vi "拉压判定.vi"(7 "Result":refnum<vi>, 10 "判定参数":T2, 11 "XY曲线":cluster{"X":dbl[], "Y":dbl[]}[](array[cluster])) -> (2 "大小":i32, 3 "OK？":bool)   [LabVIEW 2020]
panel:
  in  "最大值判定":T1
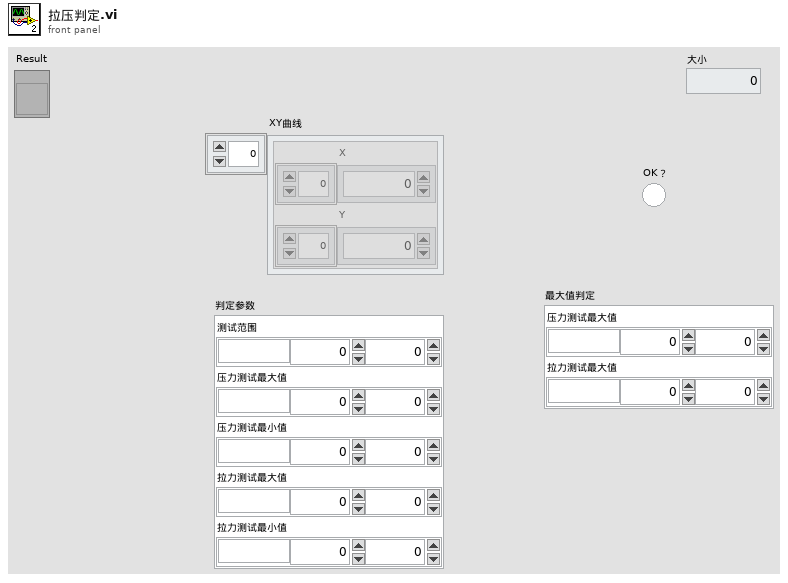
[diagram p1: front panel]
types:
  T1 = cluster{"压力测试最大值":cluster{"单位":string, "下限":dbl, "上限":dbl}, "拉力测试最大值":cluster{"单位":string, "下限":dbl, "上限":dbl}}
  T2 = cluster{"测试范围":cluster{"单位":string, "下限":dbl, "上限":dbl}, "压力测试最大值":cluster{"单位":string, "下限":dbl, "上限":dbl}, "压力测试最小值":cluster{"单位":string, "下限":dbl, "上限":dbl}, "拉力测试最大值":cluster{"单位":string, "下限":dbl, "上限":dbl}, "拉力测试最小值":cluster{"单位":string, "下限":dbl, "上限":dbl}}
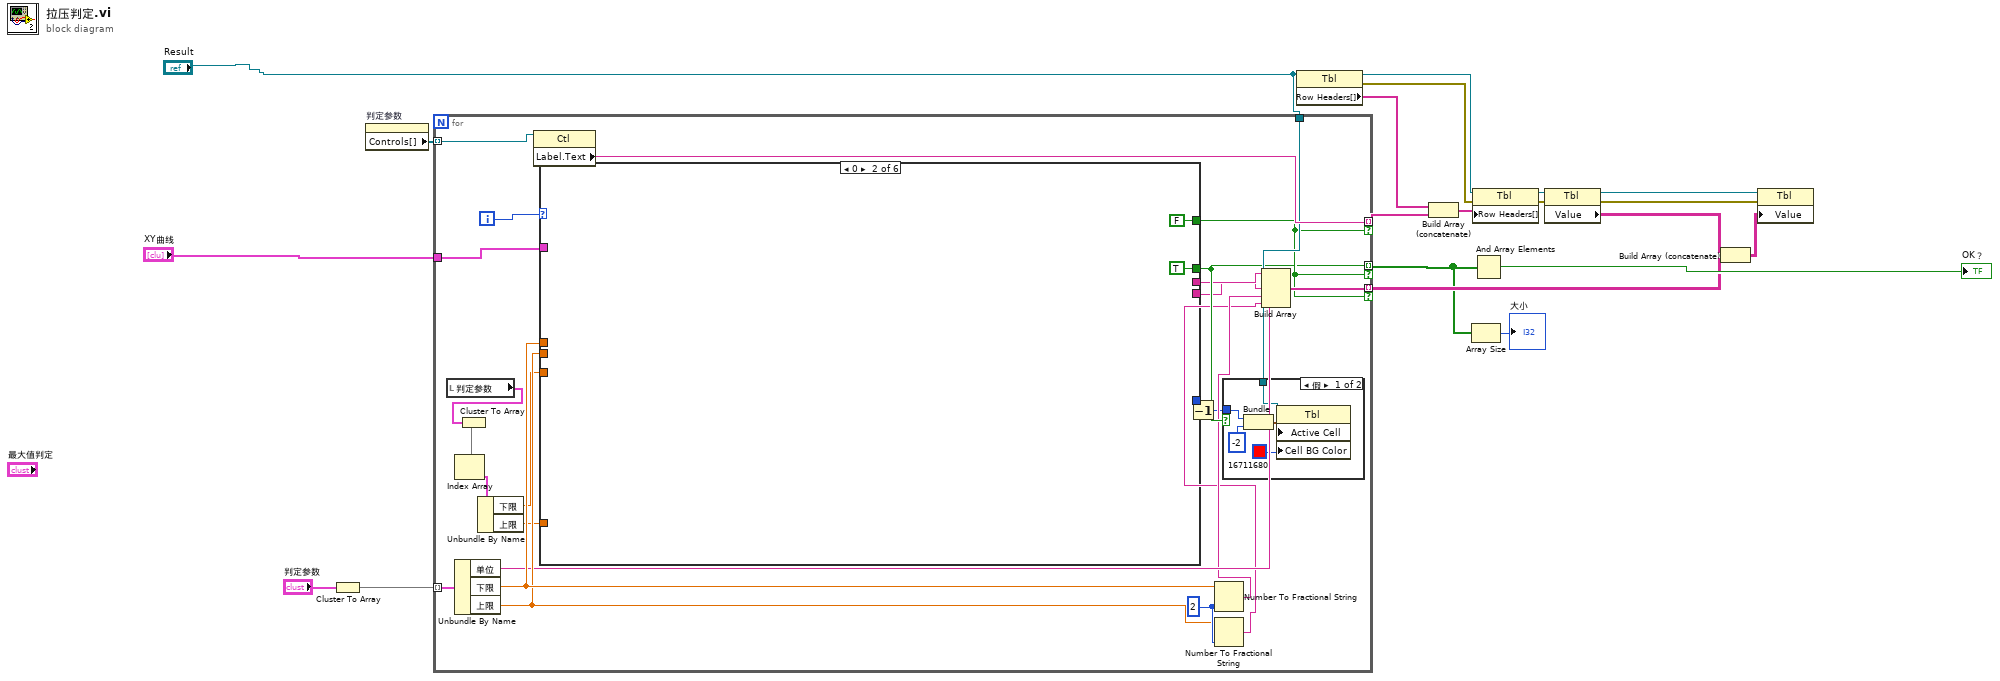
[diagram p0: block diagram]
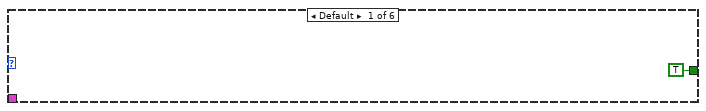
[diagram p3: hidden frame]
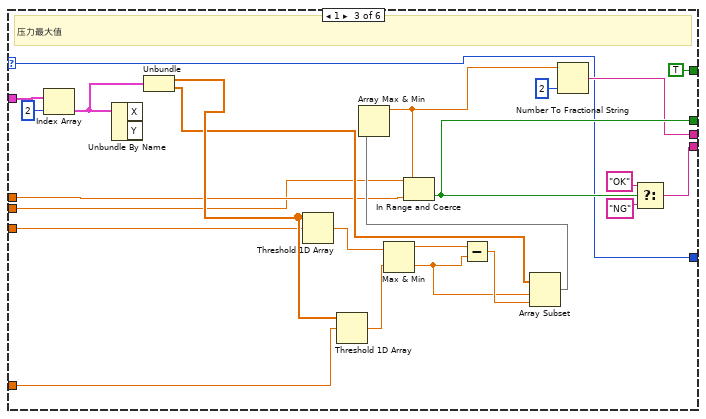
[diagram p4: hidden frame]
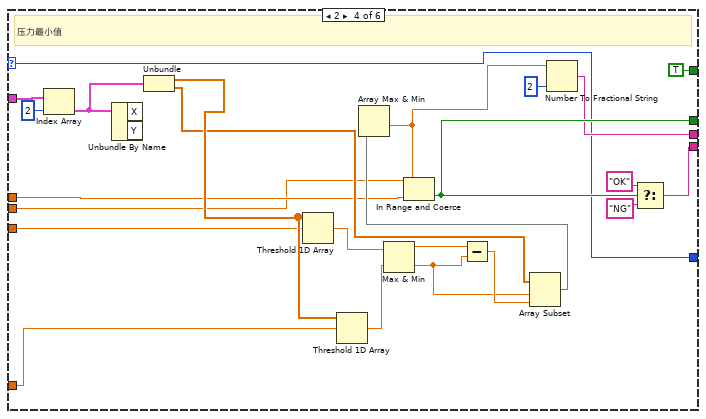
[diagram p5: hidden frame]
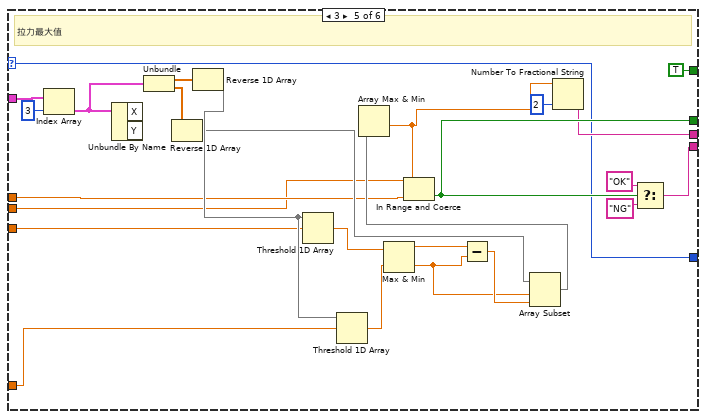
[diagram p6: hidden frame]
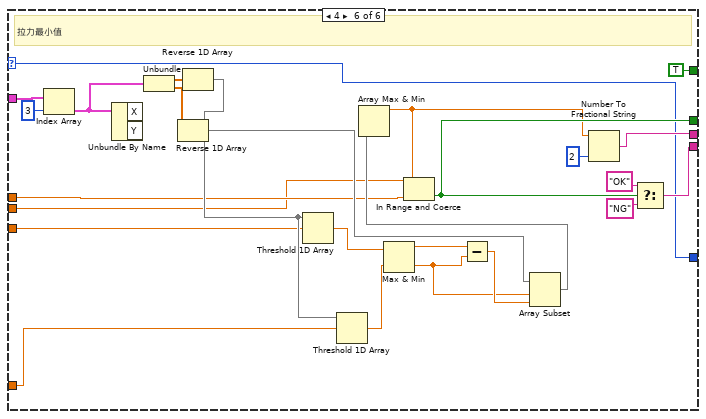
[diagram p7: hidden frame]
diagram:
  n1 = Cluster To Array(cluster="判定参数") -> (array=w20:cluster{"单位":string, "下限":dbl, "上限":dbl}[])
  n2 = property on="判定参数" class="Clust (严格)"() -> ("Controls[]"=w18:refnum<vi>[])  [unwired: 2 in, 2 out]
  n3 = for {
    tunnel: w20 -> [w44] mode=indexing
    tunnel: w18 -> [w42] mode=indexing
    tunnel: "XY曲线" -> [w41]
    tunnel: [w32] -> w2 mode=indexing if=w34
    tunnel: [w37] -> w4 mode=indexing if=w34
    tunnel: [w36] -> w6 mode=indexing if=w34
    tunnel: "Result" -> [w35]
    i -> [w43]
    w40 = i16 2 ("精度(6)")
    n4 = local read "判定参数"() -> (w26:T2)
    n5 = Unbundle By Name(w44) -> ("单位"=w30:string, "下限"=w39:dbl, "上限"=w38:dbl)
    n6 = Cluster To Array(cluster=w26) -> (array=w25:cluster{"单位":string, "下限":dbl, "上限":dbl}[])
    n7 = Index Array(array=w25) -> (element=w24:cluster{"单位":string, "下限":dbl, "上限":dbl})  [unwired: 1 in]
    n8 = Unbundle By Name(w24) -> ("下限"=w23:dbl, "上限"=w22:dbl)
    n9 = property class="Ctl"(reference=w42) -> ("Label.Text"=w36:string)  [unwired: 1 in, 2 out]
    n10 = case shown="0" w43 {
      selector: w43 -> [_ _ w57 w81 w108 w134]
      tunnel: w41 -> [_ _ w76 w100 w126 w152]
      tunnel: [_ _ w73 w97 w123 w149] -> w29
      tunnel: [_ TRUE w72 w96 w122 w148] -> w32
      tunnel: w39 -> [_ _ w56 w80 w104 w130]
      tunnel: w38 -> [_ _ w55 w79 w103 w129]
      tunnel: [TRUE FALSE TRUE TRUE TRUE TRUE] -> w34
      tunnel: [_ _ w58 w82 w109 w136] -> w31
      tunnel: [_ _ w57 w81 w108 w134] -> w33
      tunnel: w23 -> [_ _ w54 w78 w102 w128]
      tunnel: w22 -> [_ _ w53 w77 w101 w127]
      frame Default {
      }
      frame 0 {
      }
      frame 1 {
        # "压力最大值"
        n11 = Index Array(array=w76, index=2 ("索引")) -> (element=w67:cluster{"X":dbl[], "Y":dbl[]})
        n12 = Unbundle By Name(w67) -> ()  [unwired: 2 out]
        n13 = Unbundle(w67) -> ("X"=w66:dbl[], "Y"=w63:dbl[])
        n14 = Threshold 1D Array(2:w54, 3:w66) -> (0:w70:dbl)  [unwired: 1 in]
        n15 = Threshold 1D Array(2:w53, 3:w66) -> (0:w69:dbl)  [unwired: 1 in]
        n16 = Max & Min(x=w70, y=w69) -> (max(x,y)=w68:dbl, min(x,y)=w64:dbl)
        n17 = Subtract(x=w68, y=w64) -> (x-y=w65:dbl)
        n18 = Array Subset(array=w63, index=w64, length=w65) -> (w62:dbl[])
        n19 = Array Max & Min(array=w62) -> (max value=w59:dbl)  [unwired: 3 out]
        n20 = In Range and Coerce(upper limit=w55, x=w59, lower limit=w56) -> (In Range?=w72:bool)  [unwired: 1 out]
        n21 = Number To Fractional String(number=w59, precision (6)=i16 2 ("精度(6)")) -> (F-format string=w58:string)  [unwired: 2 in]
        n22 = Select(t="OK", s=w72, f="NG") -> (s? t:f=w73:string)
      }
      frame 2 {
        # "压力最小值"
        n23 = Index Array(array=w100, index=2 ("索引")) -> (element=w91:cluster{"X":dbl[], "Y":dbl[]})
        n24 = Unbundle By Name(w91) -> ()  [unwired: 2 out]
        n25 = Unbundle(w91) -> ("X"=w90:dbl[], "Y"=w87:dbl[])
        n26 = Threshold 1D Array(2:w78, 3:w90) -> (0:w94:dbl)  [unwired: 1 in]
        n27 = Threshold 1D Array(2:w77, 3:w90) -> (0:w93:dbl)  [unwired: 1 in]
        n28 = Max & Min(x=w94, y=w93) -> (max(x,y)=w92:dbl, min(x,y)=w88:dbl)
        n29 = Subtract(x=w92, y=w88) -> (x-y=w89:dbl)
        n30 = Array Subset(array=w87, index=w88, length=w89) -> (w86:dbl[])
        n31 = Array Max & Min(array=w86) -> (min value=w83:dbl)  [unwired: 3 out]
        n32 = In Range and Coerce(upper limit=w79, x=w83, lower limit=w80) -> (In Range?=w96:bool)  [unwired: 1 out]
        n33 = Number To Fractional String(number=w83, precision (6)=i16 2 ("精度(6)")) -> (F-format string=w82:string)  [unwired: 2 in]
        n34 = Select(t="OK", s=w96, f="NG") -> (s? t:f=w97:string)
      }
      frame 3 {
        # "拉力最大值"
        n35 = Index Array(array=w126, index=3 ("索引")) -> (element=w117:cluster{"X":dbl[], "Y":dbl[]})
        n36 = Unbundle By Name(w117) -> ()  [unwired: 2 out]
        n37 = Unbundle(w117) -> ("X"=w116:dbl[], "Y"=w113:dbl[])
        n38 = Reverse 1D Array(array=w113) -> (reversed array=w106:dbl[])
        n39 = Reverse 1D Array(array=w116) -> (reversed array=w107:dbl[])
        n40 = Threshold 1D Array(2:w102, 3:w107) -> (0:w120:dbl)  [unwired: 1 in]
        n41 = Threshold 1D Array(2:w101, 3:w107) -> (0:w119:dbl)  [unwired: 1 in]
        n42 = Max & Min(x=w120, y=w119) -> (max(x,y)=w118:dbl, min(x,y)=w114:dbl)
        n43 = Subtract(x=w118, y=w114) -> (x-y=w115:dbl)
        n44 = Array Subset(array=w106, index=w114, length=w115) -> (w112:dbl[])
        n45 = Array Max & Min(array=w112) -> (min value=w111:dbl)  [unwired: 3 out]
        n46 = In Range and Coerce(upper limit=w103, x=w111, lower limit=w104) -> (In Range?=w122:bool)  [unwired: 1 out]
        n47 = Number To Fractional String(number=w111, precision (6)=i16 2 ("精度(6)")) -> (F-format string=w109:string)  [unwired: 2 in]
        n48 = Select(t="OK", s=w122, f="NG") -> (s? t:f=w123:string)
      }
      frame 4 {
        # "拉力最小值"
        n49 = Index Array(array=w152, index=3 ("索引")) -> (element=w143:cluster{"X":dbl[], "Y":dbl[]})
        n50 = Unbundle By Name(w143) -> ()  [unwired: 2 out]
        n51 = Unbundle(w143) -> ("X"=w142:dbl[], "Y"=w139:dbl[])
        n52 = Reverse 1D Array(array=w139) -> (reversed array=w132:dbl[])
        n53 = Reverse 1D Array(array=w142) -> (reversed array=w133:dbl[])
        n54 = Threshold 1D Array(2:w128, 3:w133) -> (0:w146:dbl)  [unwired: 1 in]
        n55 = Threshold 1D Array(2:w127, 3:w133) -> (0:w145:dbl)  [unwired: 1 in]
        n56 = Max & Min(x=w146, y=w145) -> (max(x,y)=w144:dbl, min(x,y)=w140:dbl)
        n57 = Subtract(x=w144, y=w140) -> (x-y=w141:dbl)
        n58 = Array Subset(array=w132, index=w140, length=w141) -> (w138:dbl[])
        n59 = Array Max & Min(array=w138) -> (max value=w135:dbl)  [unwired: 3 out]
        n60 = In Range and Coerce(upper limit=w129, x=w135, lower limit=w130) -> (In Range?=w148:bool)  [unwired: 1 out]
        n61 = Number To Fractional String(number=w135, precision (6)=i16 2 ("精度(6)")) -> (F-format string=w136:string)  [unwired: 2 in]
        n62 = Select(t="OK", s=w148, f="NG") -> (s? t:f=w149:string)
      }
    }
    n63 = Decrement(x=w33) -> (x-1=w21:i32)
    n64 = Number To Fractional String(number=w39, precision (6)=w40) -> (F-format string=w28:string)  [unwired: 2 in]
    n65 = Number To Fractional String(number=w38, precision (6)=w40) -> (F-format string=w27:string)  [unwired: 2 in]
    n66 = case shown="假" w32 {
      tunnel: w35 -> [w49 _]
      tunnel: w21 -> [w45 _]
      frame False {
        n67 = Bundle(w45, -2) -> (w47:cluster{i32, i32})  [unwired: 1 in]
        n68 = property class="Tbl"(reference=w49, "Active Cell"=w47, "Cell BG Color"=u32 16711680 ("活动单元格:单元格背景色")) -> ()  [unwired: 1 in, 2 out]
      }
      frame True {
      }
    }
    n69 = Build Array(w31, w30, w29, w28, w27) -> (w37:string[])
  }
  n70 = property class="Tbl"(reference="Result") -> (reference out=w8:refnum<vi>, error out=w13:errorcluster, "Row Headers[]"=w5:string[])  [unwired: 1 in]
  n71 = Build Array (concatenate)(w5, w6) -> (w7:string[])
  n72 = Array Size(array=w2) -> (size(s)=→"大小":i32)
  n73 = property class="Tbl"(reference=w8, error in=w13, "Row Headers[]"=w7) -> (reference out=w9:refnum<vi>, error out=w12:errorcluster)
  n74 = And Array Elements(Boolean array=w2) -> (logical AND=→"OK？":bool)
  n75 = property class="Tbl"(reference=w9, error in=w12) -> (reference out=w10:refnum<vi>, error out=w11:errorcluster, "Value"=w14:string[][])
  n76 = Build Array (concatenate)(w14, w4) -> (w15:string[][])
  n77 = property class="Tbl"(reference=w10, error in=w11, "Value"=w15) -> ()  [unwired: 2 out]
